vi "Send S&E Alarm Analog message.vi"(2 "Send(T)":bool=TRUE, 7 "S&E Alarm":T1, 9 "error in (no error)":errorcluster, 12 "Loc Sub ID/Alarm ID":u16, 13 "Elevated priority":bool) -> (6 "Loop ID out":u16, 10 "error out":errorcluster)   [LabVIEW 2011]
doc: "Put error message in the S&E Q. CAn also send if no error, debends exclusively on boolean in."
uses:
  S&E Analog Alarm type.ctl
  GUI/Status Indikator Helper.ctl
  emi Lib/System 01/0 - General/S&E reporting/Private/_emi_ S&E Message.ctl
  emi Lib/System 01/0 - General/S&E reporting/Private/_emi_ S&E Message type.ctl
  emi Lib/System 01/0 - General/Private/_emi_GFV System ID.vi
panel:
  in  "Loop ID in(No Loop)":u16=9999
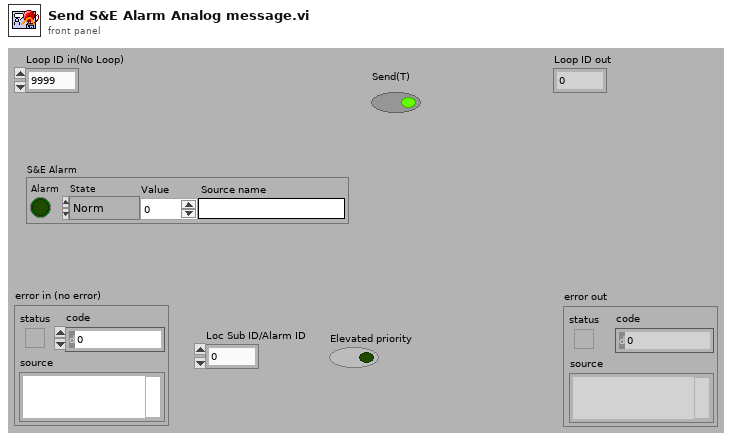
[diagram p1: front panel]
types:
  T1 = typedef "S&E Analog Alarm type.ctl" = cluster{"Alarm":bool, "State":T2, "Value":dbl, "Source name":string}
  T2 = typedef "Status Indikator Helper.ctl" = enum16{"Norm", "L", "H", "LL", "HH", "Value", "Technical"}
  T3 = typedef "_emi_ S&E Message type.ctl" = enum16{"Error/Warning", "Note", "Debug", "Event", "Alarm Analog", "Alarm Digital", "Annotation"}
  T4 = typedef "_emi_ S&E Message.ctl" = cluster{"Type":T3, "Originate time":dbl, "System":u8, "Loop":u16, "Sub ID":u16, "Elevated priority":bool, "E&S Message content":variant}
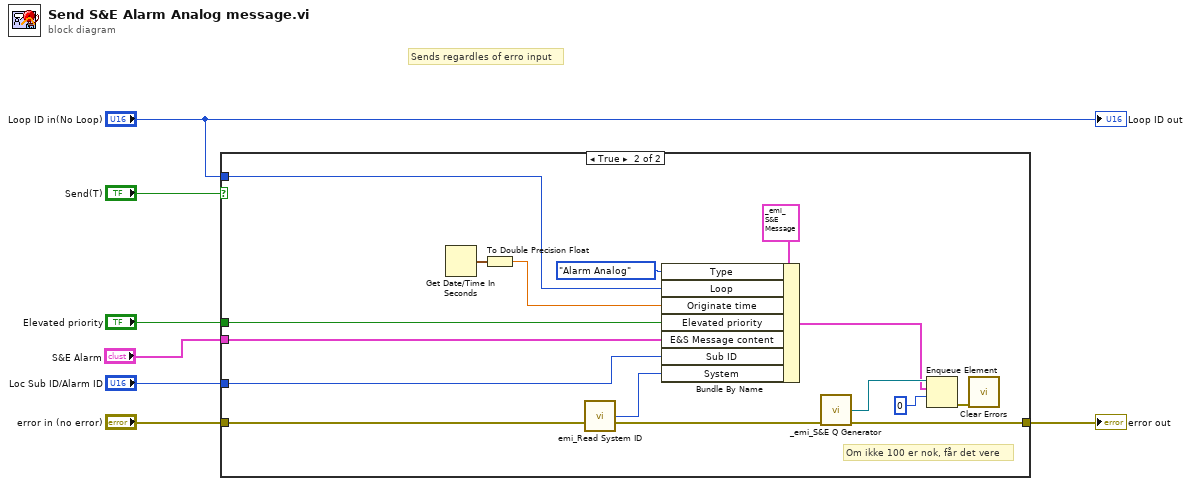
[diagram p0: block diagram]
diagram:
  # "Sends regardles of erro input"
  n1 = case shown="True" "Send(T)" {
    tunnel: "Loop ID in(No Loop)" -> [_ w20]
    tunnel: "Elevated priority" -> [_ w21]
    tunnel: "error in (no error)" -> [w8 w12]
    tunnel: [w8 w18] -> w4
    tunnel: "Loc Sub ID/Alarm ID" -> [_ w14]
    tunnel: "S&E Alarm" -> [_ w9]
    frame False {
    }
    frame True {
      # "Om ikke 100 er nok, får det vere"
      n2 = Get Date/Time In Seconds() -> (seconds since 1Jan1904=w22:timestamp)
      n3 = To Double Precision Float(number=w22) -> (double precision float=w23:dbl)
      n4 = call "emi_Read System ID.vi"("error in (no error)"=w12) -> ("System ID"=w10:u8, "error out"=w11:errorcluster)  [unwired: 13 in]
      n5 = Bundle By Name(cluster=T4 {"Type"=enum."Error/Warning", "Originate time"=0.0, "System"=0, "Loop"=0, "Sub ID"=0, "Elevated priority"=FALSE, "E&S Message content"=variant} ("E&S Message"), "Type"=_emi__S&E_Message_type."Alarm Analog", "Loop"=w20, "Originate time"=w23, "Elevated priority"=w21, "E&S Message content"=w9, "Sub ID"=w14, "System"=w10) -> (w16:T4)
      n6 = call "_emi_S&E Q Generator.vi"("error in (no error)"=w11) -> ("E&S Message Q"=w17:refnum<queue>, "error out"=w18:errorcluster)  [unwired: 13 in]
      n7 = Enqueue Element(queue=w17, element=w16, timeout in ms (-1)=0) -> (error out=w13:errorcluster)  [unwired: 1 in, 2 out]
      n8 = call <vilib>:"Clear Errors.vi"("error in (no error)"=w13) -> ()  [unwired: 6 in, 1 out]
    }
  }
  "error out" <- w4
  "Loop ID out" <- "Loop ID in(No Loop)"
